vi "Thorlabs FW102C Read & Write demo.vi"() -> ()   [LabVIEW 2011]
doc: "This example shows how to acquire a power measurement using the VIs of the driver."
uses:
  <instrlib>/Thorlabs_FW102C/Thorlabs_FW102C.lvlib
panel:
  out "Sensor Mode":T1(ring)
  out "COM Ports":string[](array[string])
  out "Position get":i32
  in  "Position set":i32=5
  out "Speed":enum16{"Slow Speed", "High Speed"}(ring)
  out "Trigger Mode":enum16{"Input Mode", "Output Mode"}(ring)
  out "Position Count":i32
  out "ID":string
  # "(c) 2015 <Thorlabs>.  ALL RIGHTS RESERVED."
  # "Connect"
  # "Set data"
  # "Read data"
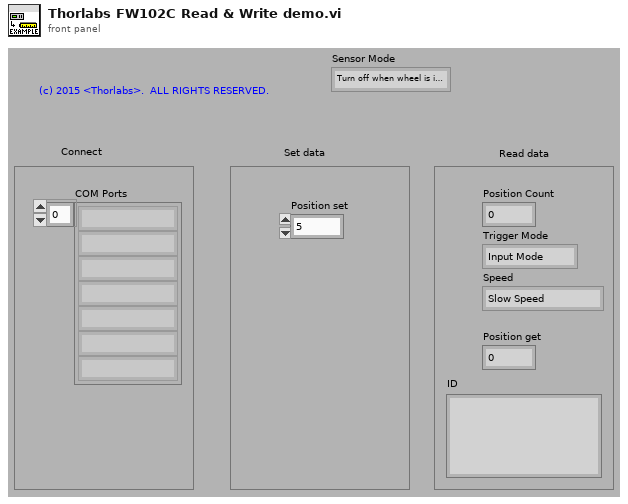
[diagram p1: front panel]
types:
  T1 = enum16{"Turn off when wheel is idle to eliminate stray light", "Remain active"}
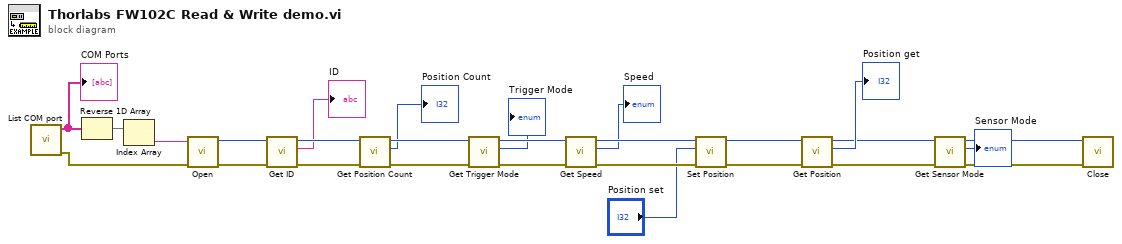
[diagram p0: block diagram]
diagram:
  n1 = call <instrlib>:"List COM port.vi"() -> ("error out"=w22:errorcluster, "COM Ports"=w25:string[])  [unwired: 10 in]
  "COM Ports" <- w25
  n2 = Reverse 1D Array(array=w25) -> (reversed array=w24:string[])
  n3 = Index Array(array=w24) -> (element=w23:string)  [unwired: 1 in]
  n4 = call <instrlib>:"Open.vi"("error in (no error)"=w22, "Serial Port"=w23) -> ("error out"=w26:errorcluster, "FW102C out"=w27:i32)  [unwired: 7 in, 1 out]
  n5 = call <instrlib>:"Get ID.vi"("error in (no error)"=w26, "FW102C in"=w27) -> ("error out"=w20:errorcluster, "ID"=→"ID":string, "FW102C out"=w21:i32)  [unwired: 7 in]
  n6 = call <instrlib>:"Get Position Count.vi"("error in (no error)"=w20, "FW102C in"=w21) -> ("error out"=w18:errorcluster, "Position Count"=→"Position Count":i32, "FW102C out"=w19:i32)  [unwired: 7 in]
  n7 = call <instrlib>:"Get Trigger Mode.vi"("error in (no error)"=w18, "FW102C in"=w19) -> ("error out"=w16:errorcluster, "Trigger Mode"=→"Trigger Mode":enum16{"Input Mode", "Output Mode"}, "FW102C out"=w17:i32)  [unwired: 7 in]
  n8 = call <instrlib>:"Get Speed.vi"("error in (no error)"=w16, "FW102C in"=w17) -> ("error out"=w14:errorcluster, "Speed"=→"Speed":enum16{"Slow Speed", "High Speed"}, "FW102C out"=w15:i32)  [unwired: 7 in]
  n9 = call <instrlib>:"Set Position.vi"("error in (no error)"=w14, "Position"="Position set", "FW102C in"=w15) -> ("error out"=w12:errorcluster, "FW102C out"=w13:i32)  [unwired: 7 in]
  n10 = call <instrlib>:"Get Position.vi"("error in (no error)"=w12, "FW102C in"=w13) -> ("error out"=w11:errorcluster, "Position"=→"Position get":i32, "FW102C out"=w4:i32)  [unwired: 7 in]
  n11 = call <instrlib>:"Get Sensor Mode.vi"("error in (no error)"=w11, "FW102C in"=w4) -> ("error out"=w5:errorcluster, "Sensor Mode"=→"Sensor Mode":T1, "FW102C out"=w3:i32)  [unwired: 7 in]
  n12 = call <instrlib>:"Close.vi"("error in (no error)"=w5, "FW102C in"=w3) -> ()  [unwired: 9 in, 1 out]
